vi "Write Key Path.vi"(6 "Key Name":string, 7 "Section":string, 8 "error in (no error)":errorcluster, 9 "create file if necessary (T)":bool=TRUE, 10 "Section Element":variant, 11 "Path in":path) -> (0 "error out":errorcluster, 1 "file created?":bool, 3 "Path out":path)   [LabVIEW 2024, in "Generic Config Handling.lvlib"]
doc: "This vi writes a variant to a config file.\n\nIt only accepts very basic datatypes. \n\nIt will accept 1D and 2D arrays.\n\nIf key name is not wired, then it will use the name of the section element."
uses:
  Generic Config Handling.lvlib
  <vilib>/Utility/config.llb/NI_LVConfig.lvlib
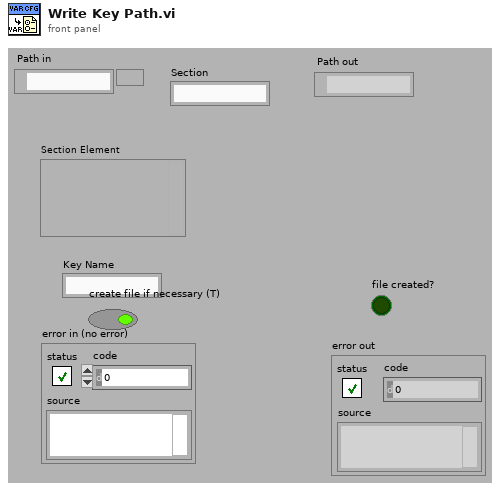
[diagram p1: front panel]
types:
  T1 = typedef "NI_LVConfig.lvlib/Config Data RefNum.ctl" = refnum<k1>
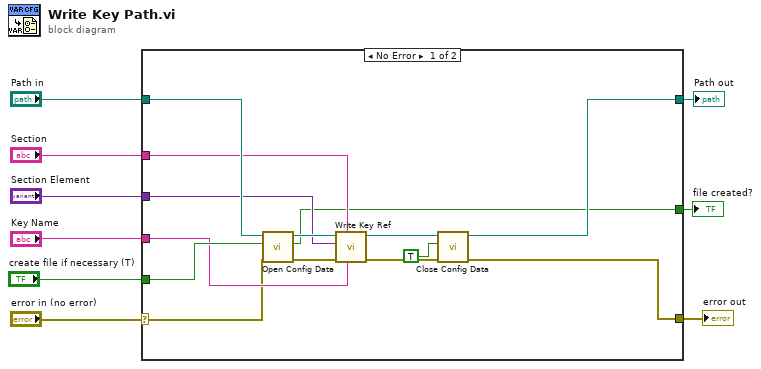
[diagram p0: block diagram]
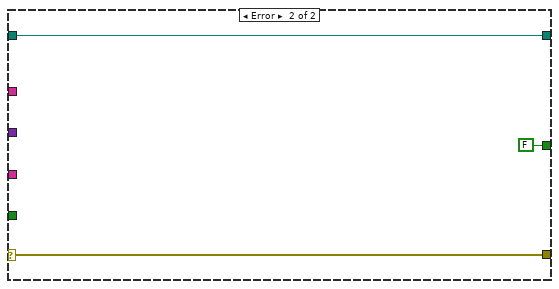
[diagram p2: hidden frame]
diagram:
  n1 = case shown="No Error" "error in (no error)" {
    selector: "error in (no error)" -> [w10 w25]
    tunnel: "Path in" -> [w22 w26]
    tunnel: [w19 w26] -> w8
    tunnel: [w18 w25] -> w7
    tunnel: "Section" -> [w15 _]
    tunnel: "Section Element" -> [w14 _]
    tunnel: "create file if necessary (T)" -> [w13 _]
    tunnel: [w12 FALSE ("file created?")] -> w3
    tunnel: "Key Name" -> [w11 _]
    frame No Error {
      n2 = call <vilib>:"Open Config Data.vi"("error in (no error)"=w10, "create file if necessary (T)"=w13, "configuration file path"=w22) -> ("error out"=w17:errorcluster, "file created?"=w12:bool, "refnum"=w21:T1)  [unwired: 6 in]
      n3 = call "Write Key Ref.vi"("Key Name"=w11, "Section"=w15, "error in (no error)"=w17, "Section Element"=w14, "Refnum in"=w21) -> ("error out"=w16:errorcluster, "Refnum out"=w20:T1)  [unwired: 5 in]
      n4 = call <vilib>:"Close Config Data.vi"("error in (no error)"=w16, "write file if changed (T)"=TRUE, "refnum"=w20) -> ("error out"=w18:errorcluster, "file path"=w19:path)  [unwired: 7 in]
    }
    frame Error {
    }
  }
  "Path out" <- w8
  "error out" <- w7
  "file created?" <- w3
